vi "Player Read Coordinates.vi"(8 "error in (no error)":errorcluster, 11 "Player in":refnum<class "Player.lvclass">) -> (0 "error out":errorcluster, 2 "Coordinates":T1[](array[typedef]), 3 "Player out":refnum<class "Player.lvclass">)   [LabVIEW 2019, in "Player.lvclass"]
uses:
  Player.lvclass
  Snake/Snake.lvclass
  Coordinate STYP.ctl
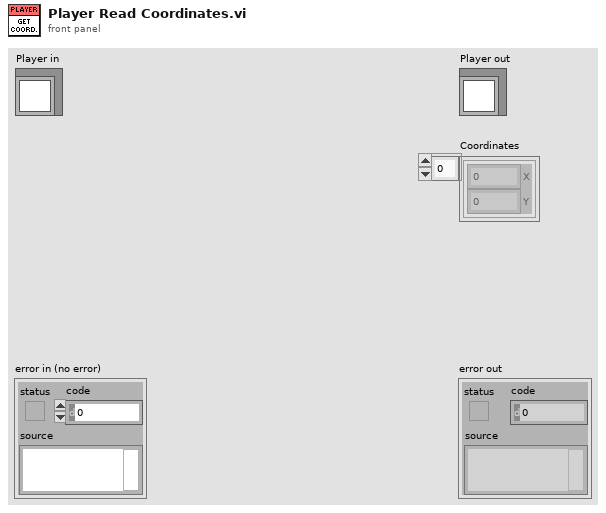
[diagram p1: front panel]
types:
  T1 = typedef "Coordinate STYP.ctl" = cluster{"X":i32, "Y":i32}
  T2 = typedef "Snake.lvclass/Snake Component STYP.ctl" = cluster{"Direction":T3, "Coordinate":T1}
  T3 = typedef "Direction STYP.ctl" = enum16{"Up", "Down", "Left", "Right"}
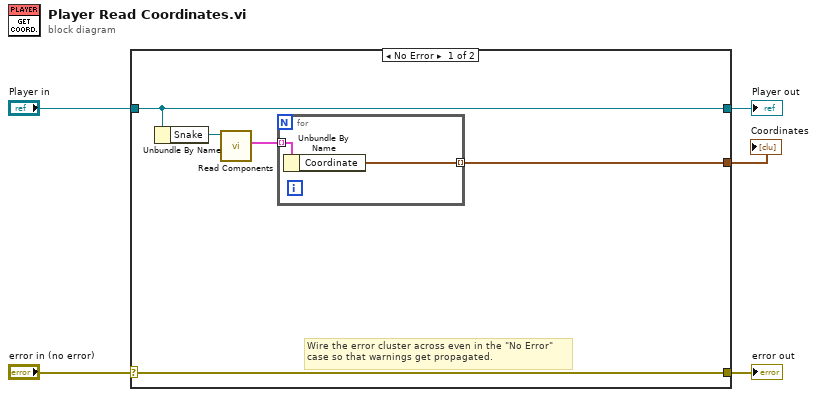
[diagram p0: block diagram]
diagram:
  n1 = case shown="No Error" "error in (no error)" {
    selector: "error in (no error)" -> [w10 w14]
    tunnel: [w10 w14] -> w4
    tunnel: [w9 w13] -> w2
    tunnel: "Player in" -> [w9 w13]
    tunnel: [w6 _] -> w1
    frame No Error {
      # "Wire the error cluster across even in the \"No Error\"\ncase so that warnings get propagated."
      n2 = Unbundle By Name(w9) -> ("Snake"=w8:refnum<class "Snake.lvclass">)
      n3 = call-dynamic "Read Components.vi"("Snake in"=w8) -> ("Components"=w7:T2[])  [unwired: 8 in, 2 out]
      n4 = for {
        tunnel: w7 -> [w12] mode=indexing
        tunnel: [w11] -> w6 mode=indexing
        n5 = Unbundle By Name(w12) -> ("Coordinate"=w11:T1)
      }
    }
    frame Error {
    }
  }
  "error out" <- w4
  "Player out" <- w2
  "Coordinates" <- w1
